vi "ConvertStringToFloat_Array-2D.vi"(7 "default value (NaN)":dbl=nan format="%#_13g", 11 "String":string[][](array[string])) -> (3 "Array of Doubles":dbl[][](array[numeric]), 5 "error in":errorcluster)   [LabVIEW 2020, in "hse-misc.lvlib"]
doc: "converts array of string values to floating point values\n\n____\nHAMPEL SOFTWARE ENGINEERING v3.8.0 (2023-12-18 14:41)"
uses:
  hse-misc.lvlib
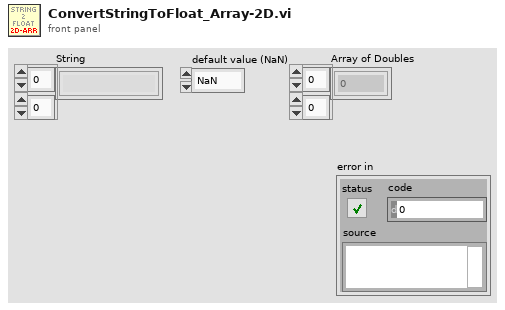
[diagram p1: front panel]
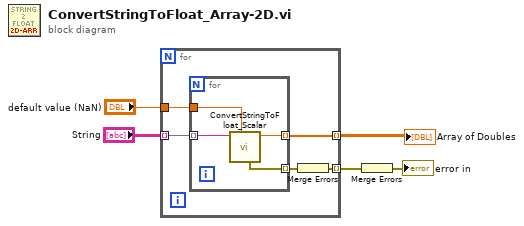
[diagram p0: block diagram]
diagram:
  n1 = for {
    tunnel: "String" -> [w10] mode=indexing
    tunnel: [w9] -> w4 mode=indexing
    tunnel: "default value (NaN)" -> [w8]
    tunnel: [w6] -> w2 mode=indexing
    n2 = for {
      tunnel: w10 -> [w14] mode=indexing
      tunnel: [w13] -> w9 mode=indexing
      tunnel: [w12] -> w7 mode=indexing
      tunnel: w8 -> [w11]
      n3 = call "ConvertStringToFloat_Scalar.vi"("default value (NaN)"=w11, "String"=w14) -> ("Double"=w13:dbl, "error out"=w12:errorcluster)  [unwired: 8 in]
    }
    n4 = Merge Errors(w7) -> (w6:errorcluster)
  }
  "Array of Doubles" <- w4
  n5 = Merge Errors(w2) -> (→"error in":errorcluster)
